vi "DBL 1D From Items.vi"(10 "Level Items":T1[](array[typedef])) -> (2 "Numeric Array":dbl[](array[numeric]))   [LabVIEW 2019]
uses:
  Ancestor Class/Front Panel Container/Tree/Tree/Type Def/Tree Item.ctl
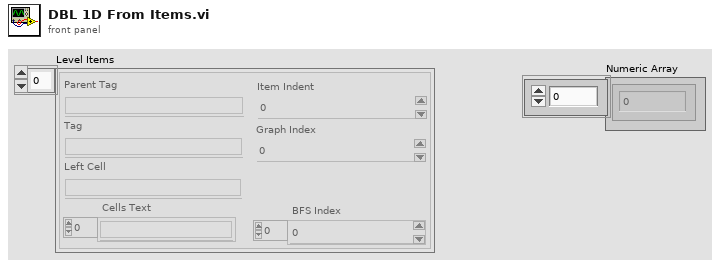
[diagram p1: front panel]
types:
  T1 = typedef "Tree Item.ctl" = cluster{"Parent Tag":string, "Tag":string, "Left Cell":string, "Cells Text":string[], "BFS Index":i32[], "Graph Index":i32, "Item Indent":i32}
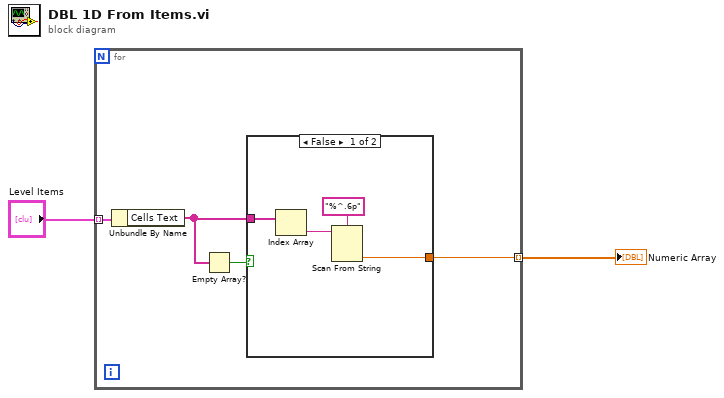
[diagram p0: block diagram]
diagram:
  n1 = for {
    tunnel: "Level Items" -> [w6] mode=indexing
    tunnel: [w5] -> w1 mode=indexing
    n2 = Unbundle By Name(w6) -> ("Cells Text"=w4:string[])
    n3 = Empty Array?(array=w4) -> (empty?=w3:bool)
    n4 = case shown="False" w3 {
      tunnel: [w8 _] -> w5
      tunnel: w4 -> [w7 _]
      frame False {
        n5 = Index Array(array=w7) -> (element=w9:string)  [unwired: 1 in]
        n6 = Scan From String(format string="%^.6p", input string=w9) -> (output 1=w8:dbl)  [unwired: 3 in, 3 out]
      }
      frame True {
      }
    }
  }
  "Numeric Array" <- w1
